vi "FTW-Ether-Construct.vi"(5 "FTW Ether Configuration":string="{\n  \"ApplicationName\": \"Featherweight Application\",\n  \"ApplicationVersion\": \"0.1.0-1\",\n  \"LoggerAddress\": \"lvq://*\",\n  \"LoggerName\": \"Log\",\n  \"LoggerDirectory\": \"[UserAppData]\\\\Featherweight\\\\Logs\",\n  \"LoggerDiskThrashDelay\": 200\n}", 11 "error in":errorcluster) -> (15 "error out":errorcluster)   [LabVIEW 2013, in "FTW-Actor.lvlib" / "FTW-Ether.lvclass"]
uses:
  FTW-Ether.lvclass
  Core/src/Reflection/FTW-Reflection-Type.vi
  Core/src/JSON/FTW-JSON-Core-LibraryFilepath.vi
  Core/src/JSON/FTW-JSON-Core-GetFlattenedValue.vi
  Core/src/JSON/FTW-JSON-Core-LibraryError.vi
  FTW-Ether-Instance.vi
  Core/utils/CodeGen/JSON Deserialize/FTW-JSON-Deserialize.xnode
  EventLogger/FTW-Logger.lvclass
panel:
  # "Inputs"
  # "Outputs"
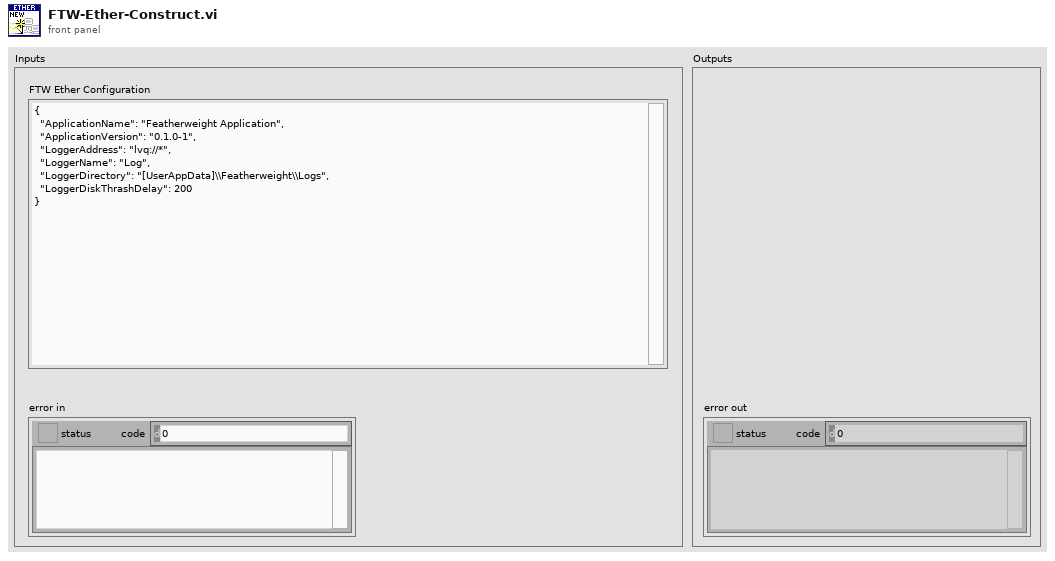
[diagram p1: front panel]
types:
  T1 = cluster{"ApplicationName":string, "ApplicationVersion":string, "LoggerAddress":string, "LoggerName":string, "LoggerDirectory":path, "LoggerDiskThrashDelay":u32}
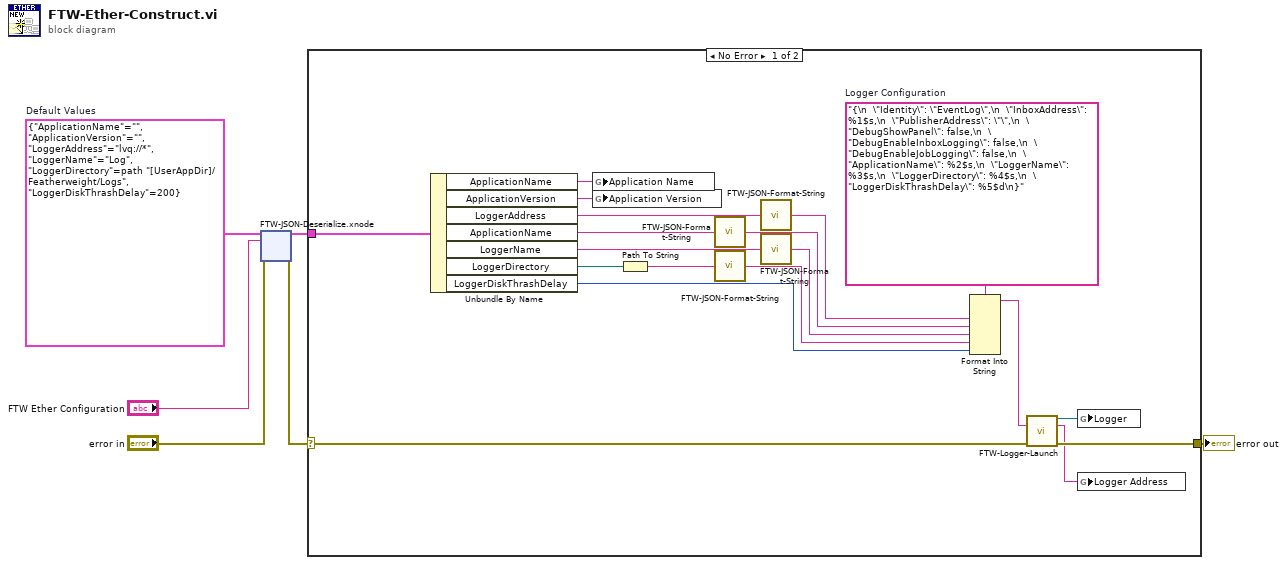
[diagram p0: block diagram]
diagram:
  w1 = T1 {"ApplicationName"="", "ApplicationVersion"="", "LoggerAddress"="lvq://*", "LoggerName"="Log", "LoggerDirectory"=path "[UserAppDir]/Featherweight/Logs", "LoggerDiskThrashDelay"=200}  # Default Values
  n1 = xnode "FTW-JSON-Deserialize.xnode"("Type and Defaults"=w1, "JSON String"="FTW Ether Configuration", "error in"="error in") -> ("Values"=w2:T1, "error out"=w3:errorcluster)
  n2 = case shown="No Error" w3 {
    selector: w3 -> [w25 w26]
    tunnel: [w24 w26] -> w6
    tunnel: w2 -> [w17 _]
    frame No Error {
      w21 = "{\n  \"Identity\": \"EventLog\",\n  \"InboxAddress\": %1$s,\n  \"PublisherAddress\": \"\",\n  \"DebugShowPanel\": false,\n  \"DebugEnableInboxLogging\": false,\n  \"DebugEnableJobLogging\": false,\n  \"ApplicationName\": %2$s,\n  \"LoggerName\": %3$s,\n  \"LoggerDirectory\": %4$s,\n  \"LoggerDiskThrashDelay\": %5$d\n}"  # Logger Configuration
      n3 = Unbundle By Name(w17) -> ("ApplicationName"=w23:string, "ApplicationVersion"=w22:string, "LoggerAddress"=w9:string, "ApplicationName"=w11:string, "LoggerName"=w13:string, "LoggerDirectory"=w15:path, "LoggerDiskThrashDelay"=w16:u32)
      n4 = global write "FTW-Ether-Instance.vi" "Application Name"(w23) -> ()
      n5 = global write "FTW-Ether-Instance.vi" "Application Version"(w22) -> ()
      n6 = Path To String(path=w15) -> (string=w7:string)
      n7 = call "FTW-JSON-Format-String.vi"("LabVIEW String"=w11) -> ("JSON String"=w10:string)
      n8 = call "FTW-JSON-Format-String.vi"("LabVIEW String"=w7) -> ("JSON String"=w14:string)
      n9 = call "FTW-JSON-Format-String.vi"("LabVIEW String"=w9) -> ("JSON String"=w8:string)
      n10 = call "FTW-JSON-Format-String.vi"("LabVIEW String"=w13) -> ("JSON String"=w12:string)
      n11 = Format Into String(format string=w21, w8, w10, w12, w14, w16) -> (resulting string=w20:string)  [unwired: 2 in, 1 out]
      n12 = call "FTW-Logger-Launch.vi"("FTW Logger Configuration"=w20, "error in"=w25) -> ("FTW Logger Connector"=w19:refnum<class "FTW-Logger.lvclass">, "Logger Address"=w18:string, "error out"=w24:errorcluster)  [unwired: 11 in]
      n13 = global write "FTW-Ether-Instance.vi" "Logger"(w19) -> ()
      n14 = global write "FTW-Ether-Instance.vi" "Logger Address"(w18) -> ()
    }
    frame Error {
    }
  }
  "error out" <- w6
